vi "Prober_MoveToXYZTheta.vi"(6 "Theta location [mdeg]":string="none", 7 "TeslaVeloxProbeStation in":refnum<class "TeslaVeloxProbeStation.lvclass">, 8 "error in (no error)":errorcluster, 9 "Z location [µm]":string="none", 10 "Y location [µm]":string="none", 11 "X location [µm]":string="none") -> (0 "error out":errorcluster, 2 "String":string, 3 "TeslaVeloxProbeStation out":refnum<class "TeslaVeloxProbeStation.lvclass">)   [LabVIEW 2018, in "TeslaVeloxProbeStation.lvclass"]
uses:
  TeslaVeloxProbeStation.lvclass
  TeslaVeloxProbeStation.lvclass/TeslaVeloxProbeStation.ctl
  Desktop/Kvasnicka/test_labview_library/Integration_toolkit_library/CascadeProbestation.lvlib
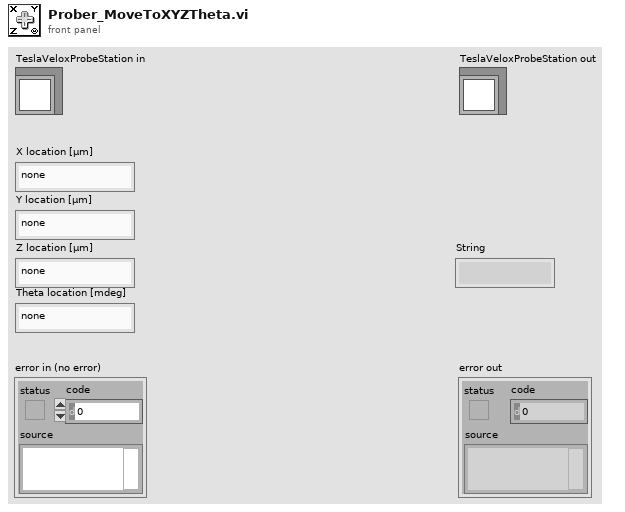
[diagram p1: front panel]
types:
  T1 = enum16{"Home", "Zero", "Center", "Current position"}
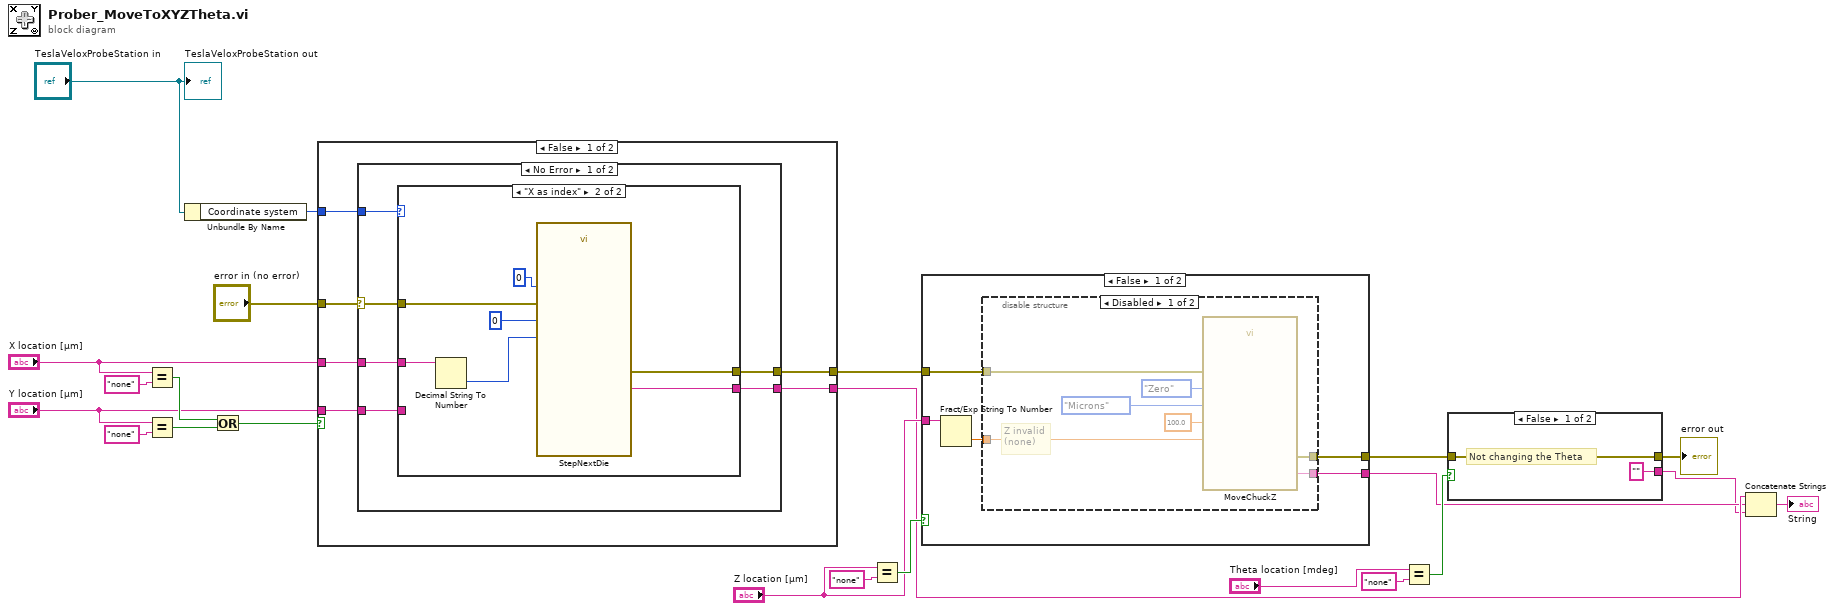
[diagram p0: block diagram]
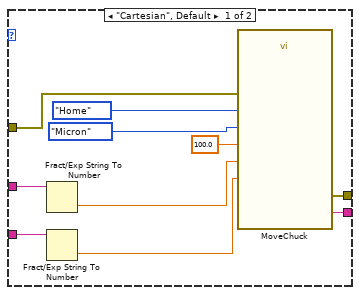
[diagram p5: hidden frame]
diagram:
  n1 = Equal?(x="X location [µm]", y="none") -> (x = y?=w23:bool)
  n2 = Equal?(x="Y location [µm]", y="none") -> (x = y?=w22:bool)
  n3 = Unbundle By Name("TeslaVeloxProbeStation in") -> ("Coordinate system"=w1:enum16{"Cartesian", "X as index"})
  n4 = Or(x=w23, y=w22) -> (x .or. y?=w21:bool)
  n5 = case shown="False" w21 {
    tunnel: "X location [µm]" -> [w29 _]
    tunnel: "Y location [µm]" -> [w28 _]
    tunnel: "error in (no error)" -> [w26 w54]
    tunnel: [w27 w54] -> w16
    tunnel: [w25 _] -> w6
    tunnel: w1 -> [w24 _]
    frame False {
      n6 = case shown="No Error" w26 {
        selector: w26 -> [w32 w53]
        tunnel: w29 -> [w35 _]
        tunnel: w28 -> [w34 _]
        tunnel: [w33 w53] -> w27
        tunnel: [w31 _] -> w25
        tunnel: w24 -> [w30 _]
        frame No Error {
          n7 = case shown="\"X as index\"" w30 {
            tunnel: w35 -> [w45 w50]
            tunnel: w34 -> [w44 _]
            tunnel: [w38 w47] -> w33
            tunnel: w32 -> [w37 w48]
            tunnel: [w36 w46] -> w31
            frame "Cartesian", Default {
              n8 = Fract/Exp String To Number(string=w45) -> (number=w43:dbl)  [unwired: 3 in, 1 out]
              n9 = Fract/Exp String To Number(string=w44) -> (number=w42:dbl)  [unwired: 3 in, 1 out]
              n10 = call "MoveChuck.vi"("X Value"=w43, "Velocity"=100.0, "Y Value"=w42, "PosRef"=T1."Home", "Unit"=enum16{"Micron", "Mils", "Index", "Jog"}."Micron", "Error In"=w37) -> ("Response"=w36:string, "Error Out"=w38:errorcluster)  [unwired: 8 in]
            }
            frame "X as index" {
              n11 = Decimal String To Number(string=w50) -> (number=w49:i32)  [unwired: 2 in, 1 out]
              n12 = call "StepNextDie.vi"("ColumnIn"=0, "RowIn"=0, "SubDieIn"=w49, "Error In"=w48) -> ("Response"=w46:string, "Error Out"=w47:errorcluster)  [unwired: 6 in, 4 out]
            }
          }
        }
        frame Error {
        }
      }
    }
    frame True {
      # "one of XY coordinate\nis invalid (none)"
    }
  }
  n13 = Equal?(x="Z location [µm]", y="none") -> (x = y?=w17:bool)
  n14 = case shown="False" w17 {
    tunnel: w16 -> [w57 w68]
    tunnel: [w56 w68] -> w13
    tunnel: "Z location [µm]" -> [w59 _]
    tunnel: [w55 _] -> w5
    frame False {
      n15 = Fract/Exp String To Number(string=w59) -> (number=w58:dbl)  [unwired: 3 in, 1 out]
      n16 = disable-structure shown="Disabled" {
        disable-tunnel: w58 -> [w66 _]
        disable-tunnel: w57 -> [w65 w67]
        disable-tunnel: [w64 w67] -> w56
        disable-tunnel: [w60 _] -> w55
        frame Disabled {
          # "Z invalid\n(none)"
          n17 = call "MoveChuckZ.vi"("Z Value"=w66, "PosRef"=enum16{"Zero", "Contact", "Current Position"}."Zero", "Unit"=enum16{"Microns", "Mils", "Jog"}."Microns", "Velocity"=100.0, "Error In"=w65) -> ("Response"=w60:string, "Error Out"=w64:errorcluster)  [unwired: 9 in]
        }
        frame Enabled {
          # "Messing with heights is not desired\nfor the tesla probestation.\nIt handles the Z heights automatically\naccording to the pre-defined z levels"
        }
      }
    }
    frame True {
    }
  }
  n18 = Equal?(x="Theta location [mdeg]", y="none") -> (x = y?=w12:bool)
  n19 = case shown="False" w12 {
    tunnel: w13 -> [w70 w71]
    tunnel: [w70 w71] -> w7
    tunnel: ["" ("String") _] -> w4
    frame False {
      # "Not changing the Theta"
    }
    frame True {
      # "Theta invalid\n(none)"
    }
  }
  "error out" <- w7
  n20 = Concatenate Strings(w6, w5, w4) -> (→"String":string)
  "TeslaVeloxProbeStation out" <- "TeslaVeloxProbeStation in"
